vi "Wavelet Packet Signal Compression.vi"() -> ()   [LabVIEW 2023]
doc: "This example shows the application of the wavelet packet decomposition in signal compression.\n\nThe wavelet packet decomposition transforms a signal into wavelet packet coefficients. The wavelet packet coefficients have most values close to zero. After quantizing the wavelet coefficients, you can set most of the coefficients to zero. So you can use entropy-based encoding techniques to reduce the bit rate of the wavelet packet coefficients and achieve signal compression. The wavelet packet-based compression method offers a more flexible analysis method than conventional wavelet transform-based methods and generates sufficient bases from which users can search for the best coefficients representation with respect to a compression objective\n\nThis example uses the WA WP Decomposition VI to transform a signal into wavelet packet coefficients and simulates the quantization for the resulting coefficients. From the quantized wavelet packet coefficients, this example reconstructs the signal using the WA WP Reconstruction VI and computes the signal to noise ratio (SNR) of the reconstructed signal. In real-world signal compression applications, you can achieve compression by using entropy-based encoding techniques such as the Huffman coding to encode the quantized wavelet packet coefficients.\n\n<b>Instructions:</b>\n1) Run this VI.\n2) Change the number of <b>Bits</b> to quantize the wavelet packet coefficients. \n3) Observe the <b>Compression Error</b> and <b>SNR (dB)</b>."
uses:
  <vilib>/addons/Wavelet Analysis/wavelet packet.llb/WA WP Decomposition (Waveform).vi
  <vilib>/addons/Wavelet Analysis/wavelet packet.llb/WA WP Reconstruction (Waveform).vi
  <vilib>/addons/_Advanced Signal Processing/NI_AdvSigProcWA.lvlib
panel:
  in  "Data":u16(ring)=117 items=["1D Example Data"=100, "-"=101, "Doppler"=102, "HOP"=103, "TF Sine"=104, "Noisy Doppler"=105, "Sea Temperature"=106, "Sp500"=107, "Power Line"=108, "Engine Knocking"=109, "HeaviSine"=110, "Bumps"=111, "Blocks"=112, "Piece Regular"=113, "HypChirps"=114, "LinChirps"=115, "Chirps"=116, "Piece Polynomial"=117, "ECG"=131, "-"=118, "2D Example Data"=119, "-"=120, "Finger Print (Image)"=121, "Iris Flower (Image)"=122, "Mammogram (Image)"=123, "Lake (Image)"=127, "Two Can 1 (Image)"=132, "Two Can 2 (Image)"=133, "Camera Man (Image)"=134]
  out "Compression Error":waveform(dbl)(graph)
  in  "Wavelet":u16(ring) items=["db02"=0, "db03"=1, "db04"=2, "db05"=3, "db06"=4, "db07"=5, "db08"=6, "db09"=7, "db10"=8, "db11"=9, "db12"=10, "db13"=11, "db14"=12, "Haar"=13, "bior1_3"=14, "bior1_5"=15, "bior2_2"=16, "bior2_4"=17, "bior2_6"=18, "bior2_8"=19, "bior3_1"=20, "bior3_3"=21, "bior3_5"=22, "bior3_7"=23, "bior3_9"=24, "bior4_4 (FBI)"=25, "bior5_5"=38, "bior6_8"=39, "coif1"=26, "coif2"=27, "coif3"=28, "coif4"=29, "coif5"=30, "sym2"=31, "sym3"=32, "sym4"=33, "sym5"=34, "sym6"=35, "sym7"=36, "sym8"=37]
  in  "stop":bool
  out "SNR (dB)":dbl
  in  "Bits":i32=8
  out "Signals":waveform(dbl)[](graph)
  # "Overview: Shows the application of the wavelet packet decomposition in signal compression.\nRequirements: LabVIEW Full Development System, Advanced Signal Processing Toolkit\nInstructions: \n1. Run this VI.\n2. Change the number of Bits to quantize the wavelet packet coefficients. \n3. Observe the Compression Error and SNR (dB).\n4. Click Stop to stop the VI."
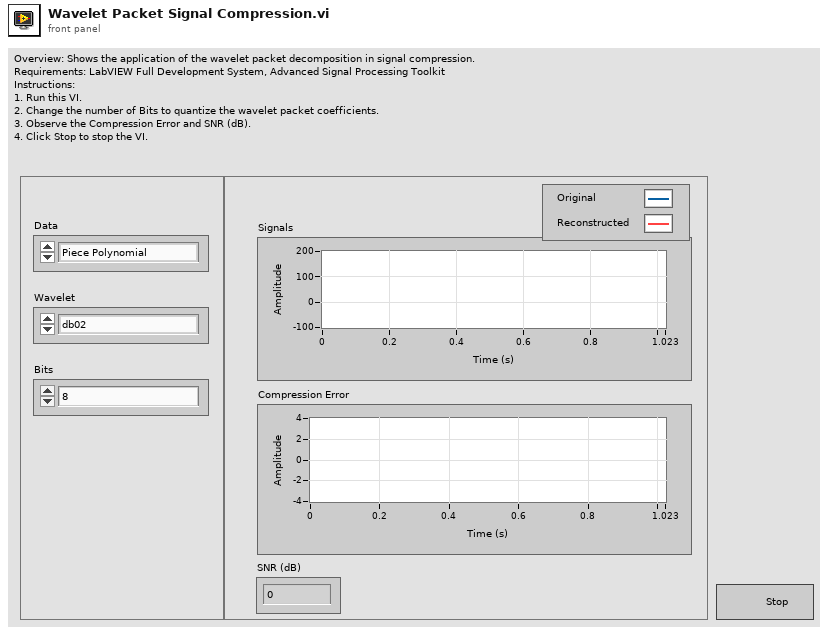
[diagram p1: front panel]
types:
  T1 = typedef "NI_AdvSigProcWA.lvlib/WA Generic Ref.ctl" = cluster{"ref":u64, "t0":timestamp, "dt":dbl}
  T2 = cluster{cluster{"lowpass":dbl[], "highpass":dbl[]}, cluster{"lowpass":dbl[], "highpass":dbl[]}}
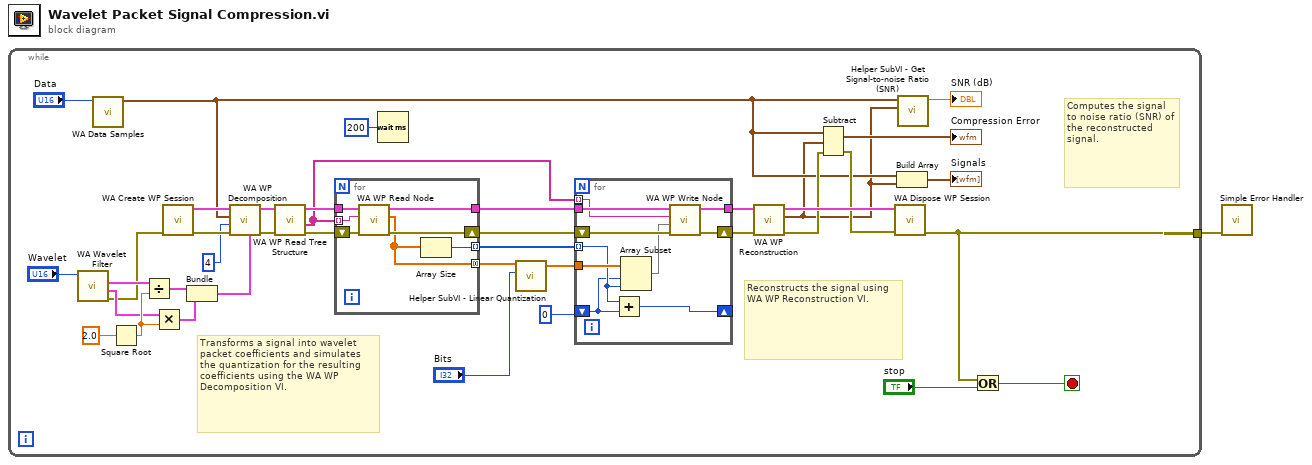
[diagram p0: block diagram]
diagram:
  n1 = while {
    tunnel: [w10] -> w1
    stop <- w15 stop-if-true
    # "Computes the signal to noise ratio (SNR) of the reconstructed signal."
    # "Reconstructs the signal using WA WP Reconstruction VI."
    # "Transforms a signal into wavelet packet coefficients and simulates the quantization for the resulting coefficients using the WA WP Decomposition VI."
    n2 = call <vilib>:"WA Wavelet Filter.vi"("wavelet"="Wavelet") -> ("error out"=w11:errorcluster, "synthesis filters"=w21:cluster{"lowpass":dbl[], "highpass":dbl[]}, "analysis filters"=w26:cluster{"lowpass":dbl[], "highpass":dbl[]})  [unwired: 3 in, 5 out]
    n3 = call <vilib>:"WA Data Samples.vi"("data"="Data") -> ("signal"=w7:waveform(dbl))  [unwired: 10 out]
    n4 = Square Root(x=2.0) -> (sqrt(x)=w24:dbl)
    n5 = Divide(x=w26, y=w24) -> (x/y=w23:cluster{"lowpass":dbl[], "highpass":dbl[]})
    n6 = Multiply(x=w21, y=w24) -> (x*y=w22:cluster{"lowpass":dbl[], "highpass":dbl[]})
    n7 = call <vilib>:"WA Create WP Session.vi"("error in (no error)"=w11) -> ("error out"=w39:errorcluster, "WP session out"=w40:T1)  [unwired: 9 out]
    n8 = Bundle(w23, w22) -> (w19:T2)  [unwired: 1 out]
    n9 = call-poly <vilib>:"WA WP Decomposition.vi"("filter banks"=w19, "error in (no error)"=w39, "levels"=4 ("level"), "signal"=w7, "WP session"=w40) -> ("error out"=w17:errorcluster, "WP session out"=w18:T1)  [unwired: 1 in, 4 out]
    n10 = call <vilib>:"WA WP Read Tree Structure.vi"("error in (no error)"=w17, "WP session"=w18) -> ("error out"=w36:errorcluster, "path"=w32:string[], "WP session out"=w37:T1)  [unwired: 7 out]
    n11 = for {
      tunnel: w37 -> [w57]
      tunnel: w32 -> [w52] mode=indexing
      shift-right: [w53] -> w34
      shift-left: w36 -> [w56]
      tunnel: [w55] -> w35
      tunnel: [w54] -> w33 mode=indexing
      tunnel: [w51] -> w2 mode=concatenating
      n12 = call <vilib>:"WA WP Read Node.vi"("error in (no error)"=w56, "path"=w52, "WP session"=w57) -> ("error out"=w53:errorcluster, "node coef"=w51:dbl[], "WP session out"=w55:T1)  [unwired: 1 in, 5 out]
      n13 = Array Size(array=w51) -> (size(s)=w54:i32)
    }
    n14 = Wait (ms)(milliseconds to wait=u32 200 ("millisecond multiple")) -> ()  [unwired: 1 out]
    n15 = call "Helper SubVI - Linear Quantization.vi"("bits"="Bits", "signal"=w2) -> ("quantized signal"=w3:dbl[])  [unwired: 9 in]
    n16 = for {
      tunnel: w35 -> [w46]
      shift-right: [w45] -> w28
      shift-left: w34 -> [w44]
      tunnel: w33 -> [w49] mode=indexing
      tunnel: w32 -> [w42] mode=indexing
      shift-right: [w47] -> _
      shift-left: 0 -> [w48]
      tunnel: w3 -> [w50]
      tunnel: [w43] -> w30
      n17 = Add(x=w49, y=w48) -> (x+y=w47:i32)
      n18 = Array Subset(array=w50, index=w48, length=w49) -> (w41:dbl[])
      n19 = call <vilib>:"WA WP Write Node.vi"("error in (no error)"=w44, "node coef"=w41, "path"=w42, "WP session"=w46) -> ("error out"=w45:errorcluster, "WP session out"=w43:T1)  [unwired: 6 out]
    }
    n20 = call-poly <vilib>:"WA WP Reconstruction.vi"("error in (no error)"=w28, "WP session"=w30) -> ("error out"=w9:errorcluster, "signal"=w6:waveform(dbl), "WP session out"=w29:T1)  [unwired: 7 out]
    n21 = Subtract(1:w6, 2:w7, 4:w9) -> (0:→"Compression Error":waveform(dbl), 3:w8:errorcluster)
    n22 = call <vilib>:"WA Dispose WP Session.vi"("error in (no error)"=w8, "WP session"=w29) -> ("error out"=w10:errorcluster)  [unwired: 9 out]
    n23 = Build Array(w7, w6) -> (→"Signals":waveform(dbl)[])
    n24 = call "Helper SubVI - Get Signal-to-noise Ratio (SNR).vi"("noisy signal"=w6, "signal"=w7) -> ("SNR (dB)"=→"SNR (dB)":dbl)  [unwired: 9 in]
    n25 = Or(x=w10, y="stop") -> (x .or. y?=w15:bool)
  }
  n26 = call <vilib>:"Simple Error Handler.vi"("error in (no error)"=w1) -> ()  [unwired: 1 in, 8 out]
